vi "chem dose flow (mLpers).vi"(4 "State":i16, 5 "Time":dbl format="%.2f", 6 "Sensor Values":dbl[](array[numeric]), 7 "Set Points":dbl[](array[numeric])) -> (0 "required data":T1={"Set Point names"=["plant flow (mL/s)", " stock concentration (mg/L)", "desired dose (mg/L)"], "required number of setpoints"=3, "required number of sensors"=0, "Sensor names"=[]}, 3 "output value":dbl)   [LabVIEW 2019]
panel:
  # "rpm/100"
  # "Enter the correct information for this control code in the required data structure below. Then make the current value default by right clicking on the border of the data structure. Select \"data operations\" and then select \"make current value default\". These values will be displayed by process controller."
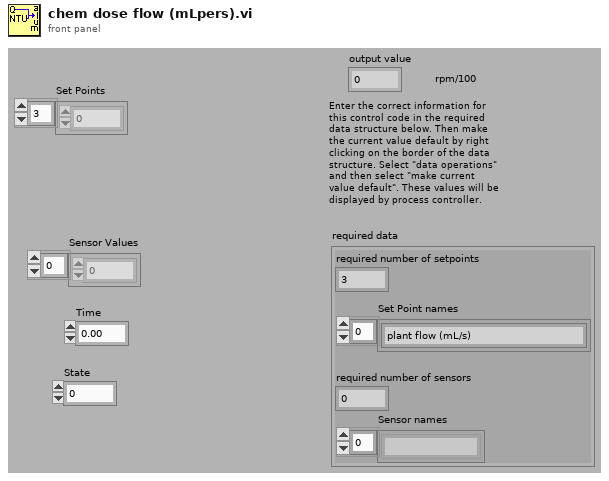
[diagram p1: front panel]
types:
  T1 = cluster{"Set Point names":string[], "required number of setpoints":u8, "required number of sensors":u8, "Sensor names":string[]}
  T2 = cluster{"Set Points[0]":dbl, "Set Points[1]":dbl, "Set Points[2]":dbl}
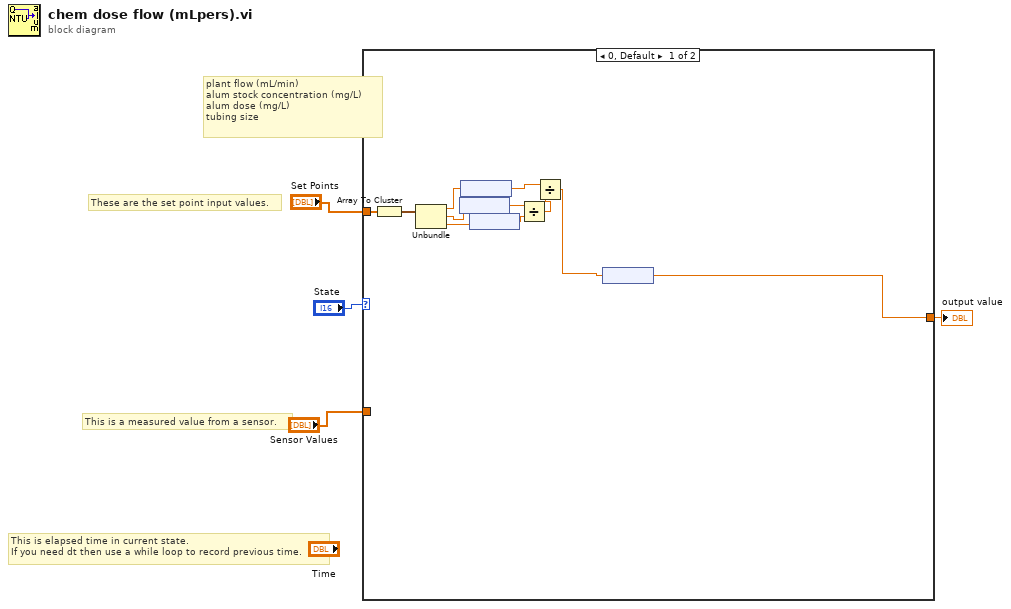
[diagram p0: block diagram]
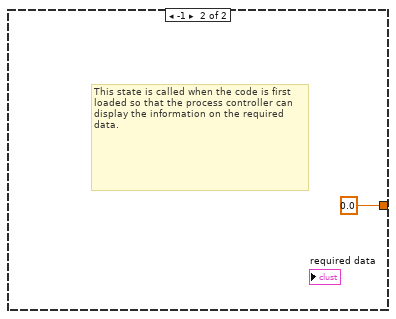
[diagram p2: hidden frame]
diagram:
  # "plant flow (mL/min)\nalum stock concentration (mg/L)\nalum dose (mg/L)\ntubing size"
  # "These are the set point input values."
  # "This is a measured value from a sensor."
  # "This is elapsed time in current state.\nIf you need dt then use a while loop to record previous time."
  n1 = case shown="0, Default" "State" {
    tunnel: [w5 0.0 ("fraction on")] -> w3
    tunnel: "Set Points" -> [w7 _]
    tunnel: "Sensor Values" -> [_ _]
    frame 0, Default {
      n2 = Array To Cluster(array=w7) -> (cluster=w15:T2)
      n3 = Unbundle(w15) -> ("Set Points[0]"=w10:dbl, "Set Points[1]"=w9:dbl, "Set Points[2]"=w8:dbl)
      n4 = node(w9) -> (w13:dbl[unit])
      n5 = node(w10) -> (w12:dbl[unit])
      n6 = node(w8) -> (w14:dbl[unit])
      n7 = Divide(x=w13, y=w14) -> (x/y=w11:dbl)
      n8 = Divide(x=w12, y=w11) -> (x/y=w6:dbl[unit])
      n9 = node(w6) -> (w5:dbl)
    }
    frame -1 {
      # "This state is called when the code is first loaded so that the process controller can display the information on the required data."
    }
  }
  "output value" <- w3
